vi "GetDeviceConstants.vi"(11 "key values":T1[](array[typedef])) -> (0 "InterPacketDelay":i32, 1 "PacketSizeKbyte":i32, 2 "MaxAttempts":i32, 3 "ReconnectInterval":dbl)   [LabVIEW 2017, in "ServerComm.lvlib"]
uses:
  <vilib>/addons/InsightCM/Devices/Shared/Common/ServerComm/ServerComm.lvlib
  <vilib>/addons/InsightCM/MessageBus/Base/controls/SectionKeyValues.ctl
  <vilib>/addons/InsightCM/MessageBus/Base/controls/KeyValuePair.ctl
  <vilib>/addons/InsightCM/Utilities/PropertyHelpers/PropertyHelpers.lvlib
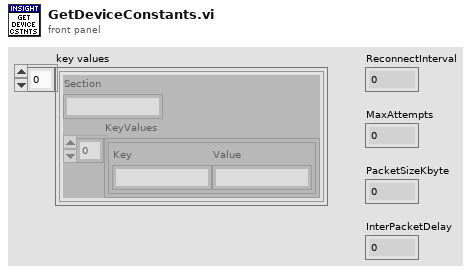
[diagram p1: front panel]
types:
  T1 = typedef "SectionKeyValues.ctl" = cluster{"Section":string, "KeyValues":T2[]}
  T2 = typedef "KeyValuePair.ctl" = cluster{"Key":string, "Value":string}
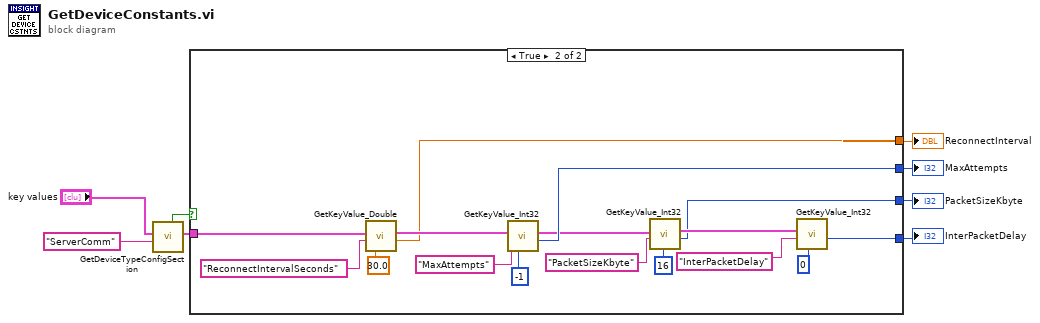
[diagram p0: block diagram]
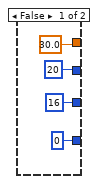
[diagram p2: hidden frame]
diagram:
  n1 = call <vilib>:"GetDeviceTypeConfigSection.vi"("key"="ServerComm", "key values"="key values") -> ("key value pairs out"=w4:T2[], "found"=w6:bool)  [unwired: 8 in]
  n2 = case shown="True" w6 {
    tunnel: w4 -> [_ w27]
    tunnel: [30.0 ("Reconnect.ReconnectInterval") w23] -> w7
    tunnel: [20 ("value") w21] -> w8
    tunnel: [16 ("value") w14] -> w2
    tunnel: [0 ("value") w13] -> w1
    frame False {
    }
    frame True {
      n3 = call <vilib>:"GetKeyValue_Double.vi"("default"=30.0 ("f"), "key"="ReconnectIntervalSeconds", "key value pairs"=w27) -> ("value"=w23:dbl, "key value pairs out"=w28:T2[])  [unwired: 6 in, 1 out]
      n4 = call <vilib>:"GetKeyValue_Int32.vi"("default"=-1 ("value"), "key"="MaxAttempts", "key value pairs"=w28) -> ("value"=w21:i32, "key value pairs out"=w18:T2[])  [unwired: 6 in, 1 out]
      n5 = call <vilib>:"GetKeyValue_Int32.vi"("default"=16 ("PacketSizeKbytes"), "key"="PacketSizeKbyte", "key value pairs"=w18) -> ("value"=w14:i32, "key value pairs out"=w17:T2[])  [unwired: 6 in, 1 out]
      n6 = call <vilib>:"GetKeyValue_Int32.vi"("default"=0 ("InterPacketDelay"), "key"="InterPacketDelay", "key value pairs"=w17) -> ("value"=w13:i32)  [unwired: 6 in, 2 out]
    }
  }
  "MaxAttempts" <- w8
  "ReconnectInterval" <- w7
  "PacketSizeKbyte" <- w2
  "InterPacketDelay" <- w1
